vi "Auto Nastawy.vi"(8 "CAN ramki in":T2 {"type" items=["CAN Data", "CAN Remote"]; "identifier" format="%.0x"}, 11 "Auto N in":cluster{T1, bool}) -> (1 "CAN konifguracyjny":T2 {"type" items=["CAN Data", "CAN Remote"]; "identifier" format="%.0x"}, 3 "Auto N out":cluster{"Sterownik in":T1, bool})   [LabVIEW 2015]
uses:
  PC/ramki konfiguracyjne.ctl
  <vilib>/RioEmbeddedCAN/RioEmbeddedCAN.llb/CANFrameControl.ctl
  Enum nastawy.ctl
panel:
  in  "TYL L":T3={"Prąd"=20.0, "Kp"=10.0, "Ki"=3.0, "OK Button"=FALSE, "ID"=2, "IDD"=3, "Sat"=250} {"Ki" format="%.1f"; "Kp" format="%.1f"; "Prąd" format="%.1f"}
  in  "SRODEK L":T3={"Prąd"=20.0, "Kp"=10.0, "Ki"=3.0, "OK Button"=FALSE, "ID"=2, "IDD"=4, "Sat"=250} {"Ki" format="%.1f"; "Kp" format="%.1f"; "Prąd" format="%.1f"}
  in  "PRZOD L":T3={"Prąd"=20.0, "Kp"=10.0, "Ki"=3.0, "OK Button"=FALSE, "ID"=2, "IDD"=2, "Sat"=250} {"Ki" format="%.1f"; "Kp" format="%.1f"; "Prąd" format="%.1f"}
  in  "TYL P":T3={"Prąd"=20.0, "Kp"=10.0, "Ki"=0.0, "OK Button"=FALSE, "ID"=1, "IDD"=3, "Sat"=250} {"Ki" format="%.1f"; "Kp" format="%.1f"; "Prąd" format="%.1f"}
  in  "SRODEK P":T3={"Prąd"=20.0, "Kp"=10.0, "Ki"=3.0000000000000013, "OK Button"=FALSE, "ID"=1, "IDD"=4, "Sat"=250} {"Ki" format="%.1f"; "Kp" format="%.1f"; "Prąd" format="%.1f"}
  in  "PRZOD P":T3={"Prąd"=20.0, "Kp"=10.000000000000004, "Ki"=3.0, "OK Button"=FALSE, "ID"=1, "IDD"=2, "Sat"=250} {"Ki" format="%.1f"; "Kp" format="%.1f"; "Prąd" format="%.1f"}
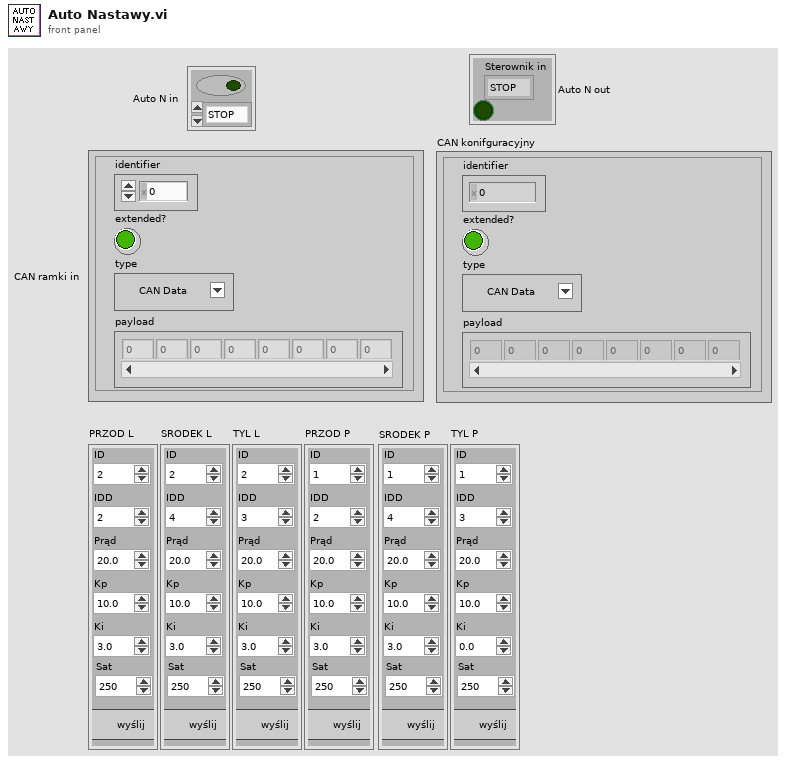
[diagram p1: front panel]
types:
  T1 = typedef "Enum nastawy.ctl" = enum16{"STOP", "PRZOD P", "SRODEK P", "TYL P", "PRZOD L", "SRODEK L", "TYL L"}
  T2 = typedef "CANFrameControl.ctl" = cluster{"identifier":u32, "extended?":bool, "type":u8, "payload":u8[]}
  T3 = typedef "ramki konfiguracyjne.ctl" = cluster{"Prąd":dbl, "Kp":dbl, "Ki":dbl, "OK Button":bool, "ID":u32, "IDD":u8, "Sat":u8}
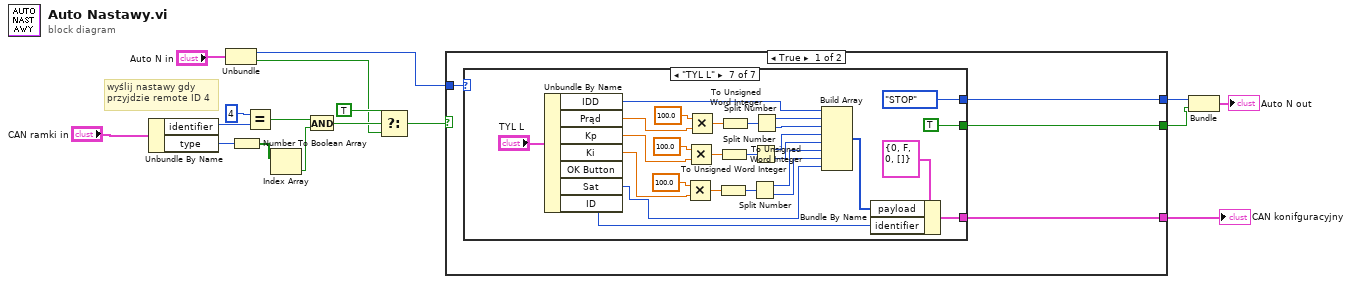
[diagram p0: block diagram]
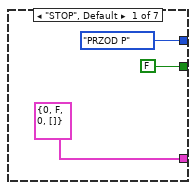
[diagram p2: hidden frame]
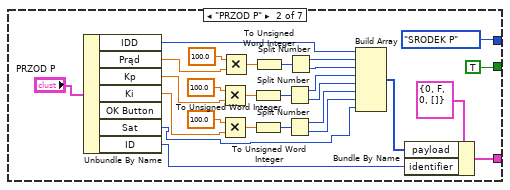
[diagram p3: hidden frame]
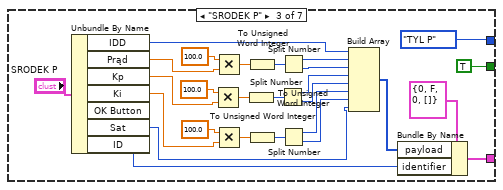
[diagram p4: hidden frame]
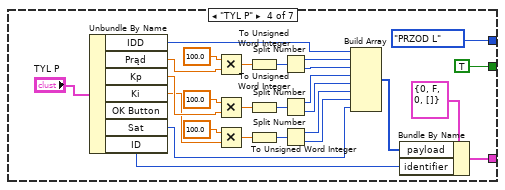
[diagram p5: hidden frame]
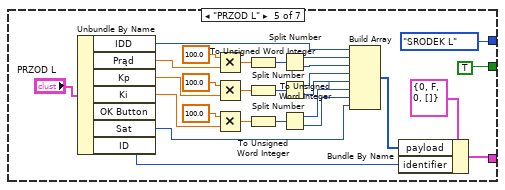
[diagram p6: hidden frame]
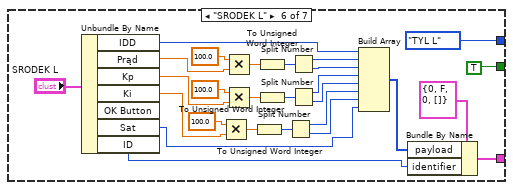
[diagram p7: hidden frame]
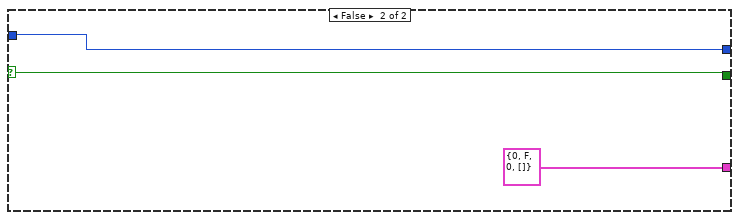
[diagram p8: hidden frame]
diagram:
  # "wyślij nastawy gdy \nprzyjdzie remote ID 4"
  n1 = Unbundle By Name("CAN ramki in") -> ("identifier"=w16:u32, "type"=w11:u8)
  n2 = Unbundle("Auto N in") -> (w2:T1, w1:bool)
  n3 = Number To Boolean Array(number=w11) -> (Boolean array=w12:bool[])
  n4 = Equal?(x=u32 4, y=w16) -> (x = y?=w15:bool)
  n5 = Index Array(array=w12) -> (element=w13:bool)  [unwired: 1 in]
  n6 = And(x=w15, y=w13) -> (x .and. y?=w14:bool)
  n7 = Select(t=TRUE, s=w14, f=w1) -> (s? t:f=w8:bool)
  n8 = case shown="True" w8 {
    selector: w8 -> [_ w187]
    tunnel: [w21 T2 {"identifier"=0, "extended?"=FALSE, "type"=0, "payload"=[]} ("CAN frame 2")] -> w17
    tunnel: w2 -> [w20 w189]
    tunnel: [w19 w189] -> w6
    tunnel: [w18 w187] -> w5
    frame True {
      n9 = case shown="\"TYL L\"" w20 {
        tunnel: [T2 {"identifier"=0, "extended?"=FALSE, "type"=0, "payload"=[]} ("CAN frame 2") w34 w61 w88 w111 w142 w169] -> w21
        tunnel: [Enum_nastawy."PRZOD P" Enum_nastawy."SRODEK P" Enum_nastawy."TYL P" Enum_nastawy."PRZOD L" Enum_nastawy."SRODEK L" Enum_nastawy."TYL L" Enum_nastawy."STOP"] -> w19
        tunnel: [FALSE TRUE TRUE TRUE TRUE TRUE TRUE] -> w18
        frame "STOP", Default {
        }
        frame "PRZOD P" {
          n10 = Unbundle By Name("PRZOD P") -> ("IDD"=w33:u8, "Prąd"=w32:dbl, "Kp"=w31:dbl, "Ki"=w30:dbl, "Sat"=w25:u8, "ID"=w26:u32)  [unwired: 1 out]
          n11 = Multiply(x=100.0, y=w31) -> (x*y=w42:dbl)
          n12 = Multiply(x=100.0, y=w30) -> (x*y=w37:dbl)
          n13 = Multiply(x=100.0, y=w32) -> (x*y=w47:dbl)
          n14 = To Unsigned Word Integer(number=w42) -> (unsigned 16bit integer=w44:u16)
          n15 = To Unsigned Word Integer(number=w37) -> (unsigned 16bit integer=w39:u16)
          n16 = To Unsigned Word Integer(number=w47) -> (unsigned 16bit integer=w50:u16)
          n17 = Split Number(x=w44) -> (hi(x)=w41:u8, lo(x)=w40:u8)
          n18 = Split Number(x=w39) -> (hi(x)=w36:u8, lo(x)=w35:u8)
          n19 = Split Number(x=w50) -> (hi(x)=w46:u8, lo(x)=w45:u8)
          n20 = Build Array(w33, w46, w45, w41, w40, w36, w35, w25) -> (w49:u8[])
          n21 = Bundle By Name(cluster=T2 {"identifier"=0, "extended?"=FALSE, "type"=0, "payload"=[]} ("CAN frame 2"), "payload"=w49, "identifier"=w26) -> (w34:T2)
        }
        frame "SRODEK P" {
          n22 = Unbundle By Name("SRODEK P") -> ("IDD"=w59:u8, "Prąd"=w58:dbl, "Kp"=w57:dbl, "Ki"=w56:dbl, "Sat"=w52:u8, "ID"=w53:u32)  [unwired: 1 out]
          n23 = Multiply(x=100.0, y=w57) -> (x*y=w69:dbl)
          n24 = Multiply(x=100.0, y=w58) -> (x*y=w74:dbl)
          n25 = Multiply(x=100.0, y=w56) -> (x*y=w64:dbl)
          n26 = To Unsigned Word Integer(number=w69) -> (unsigned 16bit integer=w71:u16)
          n27 = To Unsigned Word Integer(number=w74) -> (unsigned 16bit integer=w77:u16)
          n28 = To Unsigned Word Integer(number=w64) -> (unsigned 16bit integer=w66:u16)
          n29 = Split Number(x=w71) -> (hi(x)=w68:u8, lo(x)=w67:u8)
          n30 = Split Number(x=w77) -> (hi(x)=w73:u8, lo(x)=w72:u8)
          n31 = Split Number(x=w66) -> (hi(x)=w63:u8, lo(x)=w62:u8)
          n32 = Build Array(w59, w73, w72, w68, w67, w63, w62, w52) -> (w76:u8[])
          n33 = Bundle By Name(cluster=T2 {"identifier"=0, "extended?"=FALSE, "type"=0, "payload"=[]} ("CAN frame 2"), "payload"=w76, "identifier"=w53) -> (w61:T2)
        }
        frame "TYL P" {
          n34 = Unbundle By Name("TYL P") -> ("IDD"=w87:u8, "Prąd"=w86:dbl, "Kp"=w85:dbl, "Ki"=w84:dbl, "Sat"=w80:u8, "ID"=w79:u32)  [unwired: 1 out]
          n35 = Multiply(x=100.0, y=w86) -> (x*y=w101:dbl)
          n36 = Multiply(x=100.0, y=w85) -> (x*y=w96:dbl)
          n37 = Multiply(x=100.0, y=w84) -> (x*y=w91:dbl)
          n38 = To Unsigned Word Integer(number=w101) -> (unsigned 16bit integer=w104:u16)
          n39 = To Unsigned Word Integer(number=w96) -> (unsigned 16bit integer=w98:u16)
          n40 = To Unsigned Word Integer(number=w91) -> (unsigned 16bit integer=w93:u16)
          n41 = Split Number(x=w104) -> (hi(x)=w100:u8, lo(x)=w99:u8)
          n42 = Split Number(x=w98) -> (hi(x)=w95:u8, lo(x)=w94:u8)
          n43 = Split Number(x=w93) -> (hi(x)=w90:u8, lo(x)=w89:u8)
          n44 = Build Array(w87, w100, w99, w95, w94, w90, w89, w80) -> (w103:u8[])
          n45 = Bundle By Name(cluster=T2 {"identifier"=0, "extended?"=FALSE, "type"=0, "payload"=[]} ("CAN frame 2"), "payload"=w103, "identifier"=w79) -> (w88:T2)
        }
        frame "PRZOD L" {
          n46 = Unbundle By Name("PRZOD L") -> ("IDD"=w117:u8, "Prąd"=w118:dbl, "Kp"=w124:dbl, "Ki"=w130:dbl, "Sat"=w107:u8, "ID"=w106:u32)  [unwired: 1 out]
          n47 = Multiply(x=100.0, y=w118) -> (x*y=w116:dbl)
          n48 = Multiply(x=100.0, y=w124) -> (x*y=w123:dbl)
          n49 = Multiply(x=100.0, y=w130) -> (x*y=w129:dbl)
          n50 = To Unsigned Word Integer(number=w116) -> (unsigned 16bit integer=w113:u16)
          n51 = To Unsigned Word Integer(number=w123) -> (unsigned 16bit integer=w121:u16)
          n52 = To Unsigned Word Integer(number=w129) -> (unsigned 16bit integer=w127:u16)
          n53 = Split Number(x=w113) -> (hi(x)=w119:u8, lo(x)=w120:u8)
          n54 = Split Number(x=w121) -> (hi(x)=w125:u8, lo(x)=w126:u8)
          n55 = Split Number(x=w127) -> (hi(x)=w131:u8, lo(x)=w132:u8)
          n56 = Build Array(w117, w119, w120, w125, w126, w131, w132, w107) -> (w114:u8[])
          n57 = Bundle By Name(cluster=T2 {"identifier"=0, "extended?"=FALSE, "type"=0, "payload"=[]} ("CAN frame 2"), "payload"=w114, "identifier"=w106) -> (w111:T2)
        }
        frame "SRODEK L" {
          n58 = Unbundle By Name("SRODEK L") -> ("IDD"=w140:u8, "Prąd"=w139:dbl, "Kp"=w138:dbl, "Ki"=w137:dbl, "Sat"=w134:u8, "ID"=w133:u32)  [unwired: 1 out]
          n59 = Multiply(x=100.0, y=w137) -> (x*y=w145:dbl)
          n60 = Multiply(x=100.0, y=w139) -> (x*y=w155:dbl)
          n61 = Multiply(x=100.0, y=w138) -> (x*y=w150:dbl)
          n62 = To Unsigned Word Integer(number=w145) -> (unsigned 16bit integer=w147:u16)
          n63 = To Unsigned Word Integer(number=w155) -> (unsigned 16bit integer=w158:u16)
          n64 = To Unsigned Word Integer(number=w150) -> (unsigned 16bit integer=w152:u16)
          n65 = Split Number(x=w147) -> (hi(x)=w144:u8, lo(x)=w143:u8)
          n66 = Split Number(x=w158) -> (hi(x)=w154:u8, lo(x)=w153:u8)
          n67 = Split Number(x=w152) -> (hi(x)=w149:u8, lo(x)=w148:u8)
          n68 = Build Array(w140, w154, w153, w149, w148, w144, w143, w134) -> (w157:u8[])
          n69 = Bundle By Name(cluster=T2 {"identifier"=0, "extended?"=FALSE, "type"=0, "payload"=[]} ("CAN frame 2"), "payload"=w157, "identifier"=w133) -> (w142:T2)
        }
        frame "TYL L" {
          n70 = Unbundle By Name("TYL L") -> ("IDD"=w167:u8, "Prąd"=w166:dbl, "Kp"=w165:dbl, "Ki"=w164:dbl, "Sat"=w160:u8, "ID"=w161:u32)  [unwired: 1 out]
          n71 = Multiply(x=100.0, y=w164) -> (x*y=w172:dbl)
          n72 = Multiply(x=100.0, y=w165) -> (x*y=w177:dbl)
          n73 = Multiply(x=100.0, y=w166) -> (x*y=w182:dbl)
          n74 = To Unsigned Word Integer(number=w172) -> (unsigned 16bit integer=w174:u16)
          n75 = To Unsigned Word Integer(number=w177) -> (unsigned 16bit integer=w179:u16)
          n76 = To Unsigned Word Integer(number=w182) -> (unsigned 16bit integer=w185:u16)
          n77 = Split Number(x=w174) -> (hi(x)=w171:u8, lo(x)=w170:u8)
          n78 = Split Number(x=w179) -> (hi(x)=w176:u8, lo(x)=w175:u8)
          n79 = Split Number(x=w185) -> (hi(x)=w181:u8, lo(x)=w180:u8)
          n80 = Build Array(w167, w181, w180, w176, w175, w171, w170, w160) -> (w184:u8[])
          n81 = Bundle By Name(cluster=T2 {"identifier"=0, "extended?"=FALSE, "type"=0, "payload"=[]} ("CAN frame 2"), "payload"=w184, "identifier"=w161) -> (w169:T2)
        }
      }
    }
    frame False {
    }
  }
  "CAN konifguracyjny" <- w17
  n82 = Bundle(w6, w5) -> (→"Auto N out":cluster{T1, bool})  [unwired: 1 in]
